vi "Meas_global.vi"() -> ()   [LabVIEW 2022 SP3]
uses:
  Controls/Graph_Type.ctl
  Controls/Post_Process.ctl
  Controls/Trigger_Mode.ctl
  Controls/PWA_Data.ctl
  Controls/Correlation_cluster1.ctl
  Controls/XY_Plot_Cluster.ctl
  Controls/Time_Trace_Cluster.ctl
  Controls/Analysis_info_cluster.ctl
  Controls/Inst_type.ctl
  Controls/Instrument_Array.ctl
  Controls/channelState.ctl
  Controls/Setup.ctl
  Camera Server/Camera enum/Camera resolution.ctl
  File/File Update Cluster.ctl
  Controls/Initial Positions.ctl
  Controls/Initial Info Cluster.ctl
  Gen Trav/Multi_Run_Status.ctl
  Controls/Meas input Cluster.ctl
  Controls/portOrDev.ctl
  Controls/calType.ctl
  Controls/DAQinputType.ctl
panel:
  in  "Tab Control":T1(tab)
  in  "Delay before taking data (ms)":u32
  out "Setup complete?":bool
  in  "Status":T2
  in  "Extra Setup Ch Values":string[](array[string])
  in  "Extra Setup Ch Names":string[](array[string])
  out "Initial Info Cluster":T3[](array[typedef])
  in  "Aborted Setup":bool
  in  "Acquisition Rendezvous":T4
  in  "Time per Block (s)":dbl=100.0 format="%_4f"
  out "MeasurementEndTime":dbl format="%#.2f"
  out "MeasurementStartTime":dbl format="%#.2f"
  out "Nblocks Index":i32
  in  "Current Row Comments":string
  in  "Extra command String":string
  in  "Acquisition Ready":refnum<k4>
  out "Acq ready":bool
  out "Abs Press (mbar)":dbl=1005.0 format="%.2f"
  in  "Start Time of experiment":dbl format="%.2f"
  out "Temp":dbl=20.0 format="%.1f"
  in  "Requested No of blocks":i32
  in  "Post Process":T5
  out "Current Block No":i32
  in  "Remote control":bool
  in  "ADAM Ch Names":string[](array[string])
  in  "Processing last block?":bool
  in  "Averaging time (min)":dbl=6.0 format="%.2f"
  out "Actual Measurement time (min)":dbl=6.0 format="%.2f"
  in  "People to Email":string[](array[string])
  in  "Repeat Measurement?":bool
  in  "Blocks to Skip":i32[](array[numeric])
  in  "Iteration Number":i32
  out "OverrideWait":bool
  in  "setup":T6=enum."Show Setup"
  in  "Zero Offsetting filename":string
  out "svnRevisionOfBinaryData":u32
  out "Flattened data type":enum16{"4.x", "Standard"}(ring)
  out "Time Data was Aquired":dbl format="%.2f"
  in  "Meas Setup filename":string
  in  "Extra Comments":string
  out "ProgRevisionInfo":string
  in  "New Setup String":string
  in  "Pre Setup String":string
  in  "Comments":string
  in  "Raw data file":path
  in  "File":T7(ring)
  in  "Results file":path
  out "Raw data option":enum16{"Save raw data", "Raw data not saved"}(ring)
  out "Start of I16 data (bytes)":i64
  out "Calib file strings":string[](array[string])
  out "Calib type name":string[](array[string])
  out "DAQmx Task Name":refnum<k21>
  in  "TriggerEdge":i32(ring)=10171 items=["Rising"=10280, "Falling"=10171]
  in  "TriggerTTLsource":tag
  in  "Don't Process":bool
  in  "Acquisition Complete?":bool=TRUE
  in  "Measurement.vi Top level?":bool
  in  "Serial Port Aliases":string[][](array[string])
  in  "Called by Zero Instruments.vi":bool
  in  "DAQ Trigger Port":refnum<visa-resource-name>="COM100"
  in  "DAQ Tigger Control?":bool
  in  "Extra ADAM Channel Values":string[](array[string])
  in  "Extra ADAM Channel Names":string[](array[string])
  in  "input terminal configuration":i32(ring)=10106 items=["default"=-1, "RSE"=10083, "NRSE"=10078, "Differential"=10106, "Pseudodifferential"=12529]
  in  "Trigger mode":T8
  in  "Analogue data":enum16{"No Analogue data", "Take Analogue data"}(ring)
  in  "Time Continuous Across Blocks":bool
  in  "output polarity":u16(ring)=1 items=["do not change", "positive", "negative"]
  in  "Over/Under string":string
  in  "Acquisition_Plug_Ins to Run":string[](array[string])
  in  "PWA Data":T9
  in  "stop":bool
  in  "BSA data rate string":string
  in  "LDA data":enum16{"No LDA data", "Take LDA data"}(ring)
  in  "Use  Analogue channel to software sync with LDA":bool
  in  "Blank Output Stats for Chs":i32[](array[numeric])
  out "Initial Probe Positions":T10[](array[typedef])
  out "XYZ Positions From File":dbl[][](array[numeric])
  in  "Template File":path
  in  "Files to Update":T11[](array[typedef])
  in  "Duplicate Chs to correlate":i32[][](array[numeric]) min=0 max=8
  in  "Duplicate_Channels_by_Arithmetic":i32[][](array[numeric]) min=0 max=8
  in  "Create_Derived_Channels_by_Arithmetic":i32[][](array[numeric]) min=0 max=8
  in  "Sub Block Time (s) for Spectra and Auto Corr":dbl=1.0 min=1.0 step=1.0
  in  "Duplicate channels":i32[](array[numeric])
  in  "Smoothing setups":T12(array[cluster]) {"Y axis"."Format" items=["Decimal", "Scientific", "Engineering"]; "Y axis"."Mapping" items=["Linear", "Logarithmic"]; "X axis"."Format" items=["Decimal", "Scientific", "Engineering"]; "X axis"."Mapping" items=["Linear", "Logarithmic"]}
  in  "Cross wire + or -ve":T13(ring)
  in  "Second Graph":T15={"Plot 1"=1, "Plot 2"=3, "Save graph"=0, "Plot Type"=enum."Voltage trace"} {"Save graph" items=["Do not save plot", "Save plot"]; "Plot 2" items=["Nothing", "Velocity1", "Arr time1", "Velocity2", "Arr time2"]; "Plot 1" items=["Nothing", "Velocity1", "Arr time1", "Velocity2", "Arr time2"]}
  in  "First Graph":T15={"Plot 1"=1, "Plot 2"=3, "Save graph"=0, "Plot Type"=enum."Voltage trace"} {"Save graph" items=["Do not save plot", "Save plot"]; "Plot 2" items=["Nothing", "Velocity1", "Arr time1", "Velocity2", "Arr time2"]; "Plot 1" items=["Nothing", "Velocity1", "Arr time1", "Velocity2", "Arr time2"]}
  in  "No of bins in histogram":i32=300
  in  "correlate":i32[][](array[numeric]) min=0 max=8
  in  "Insts for plotting":u16[][](array[ring]) items=["Nothing", "Ref Prop 1", "XW1 1", "XW2 1"]
  out "Unique Times":cluster{"Time (s)":dbl[]}[](array[cluster])
  in  "Time Array Index":i32[](array[numeric])
  out "Fs Used":dbl
  in  "Analysis Info cluster":T16[](array[typedef]) {"Kurt_u" format="%_3g"; "u^4" format="%_3g"; "u^3" format="%_3g"; "Sd Error in Variance" format="%_3g"; "u^2" format="%_3g"; "Sd Error in Mean" format="%_3g"; "U" format="%_3g"; "Sync Delay Time (s)" format="%.4f"; "Total Meas Time (s)" format="%_5g"; "Skew_u" format="%_3g"; "% u'/U" format="%_3g"}
  in  "Time Trace":T20[](array[typedef])
  in  "Autocorrelation":T21[](array[typedef]) {"X array" format="%^_5g"; "Y array" format="%^_5g"}
  in  "Histogram":T21[](array[typedef]) {"X array" format="%^_5g"; "Y array" format="%^_5g"}
  in  "Spectra":T21[](array[typedef]) {"X array" format="%^_5g"; "Y array" format="%^_5g"}
  in  "Confidence Interval (%)":dbl=68.0
  in  "Timescale multiplier for independent samples":dbl=2.0
  in  "Integration threshold (0...1)":dbl=0.25
  in  "Correlation Results":T22[](array[typedef]) {"Time Window (ms)" format="%.2f"; "w^2 Paired" format="%.2f"; "u^2 Paired" format="%.2f"; "u^2w^2" format="%.2f"; "u^3w" format="%.2f"; "uw^3" format="%.2f"; "uw/u'w'" format="%.2f"; "uw^2" format="%.2f"; "u^2w" format="%.2f"; "uw" format="%.2f"}
  in  "Error Messages":string
  out "Diagnostic info":string[][](table)
  out "Vel stat display":string[][](table)
  in  "Error handler Log":string
  in  "Acquiring Pictures":bool
  in  "Webcam Overlay Text":string
  in  "Camera Resolution":T23=1 items=["Low", "Med.", "High", "Max."]
  out "Dynamically Added":T24[](array[typedef]) {"Fs" format="%#_pHz"; "syncDelay" format="%#_gms"; "Ch" min=0 step=1}
  # "The factor to multiply the integral time scale by to correct for a non-zero integration cut-off is now automatically computed using numerical function"
  # "This is the fraction of the correlation peak value at which to cut-off the integration of the correlation function"
  # "(Springer Handbook of Experimental Fluid Mechanics, eqn 23.46)"
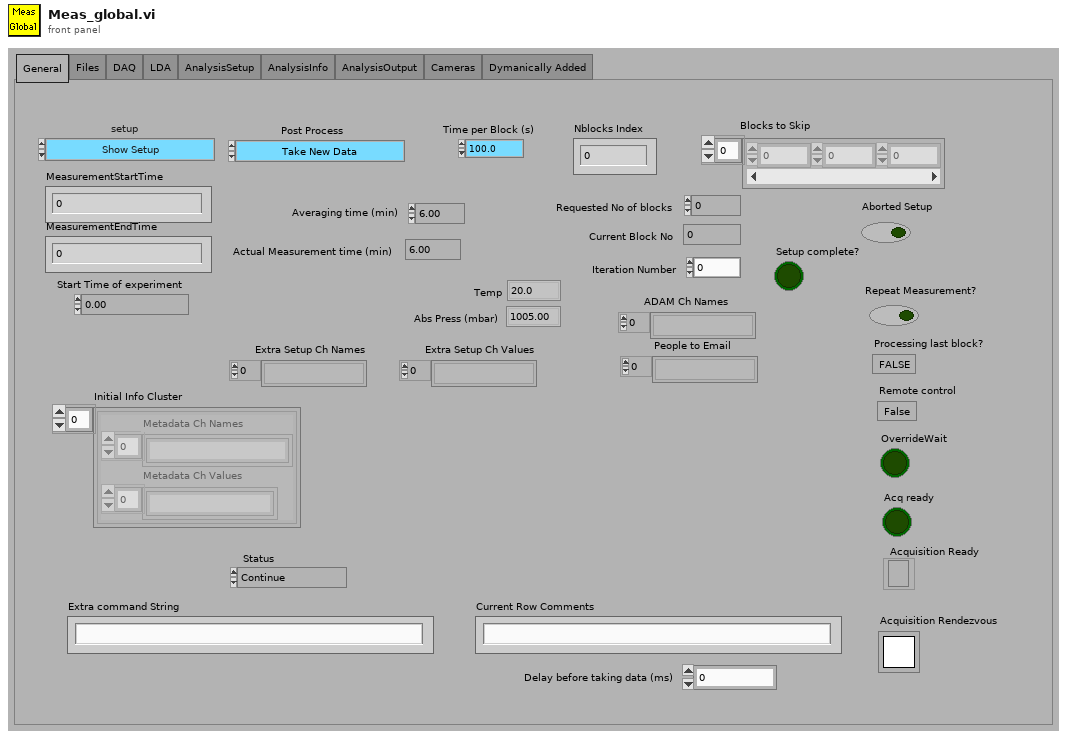
[diagram p1: front panel]
types:
  T1 = enum32{"General", "Files", "DAQ", "LDA", "AnalysisSetup", "AnalysisInfo", "AnalysisOutput", "Cameras", "Dymanically Added"}
  T2 = typedef "Multi_Run_Status.ctl" = enum16{"Continue", "Continue with Error", "Jump to Next Point", "Jump to Next Row", "Jump To Fall Back", "Terminate Run"}
  T3 = typedef "Initial Info Cluster.ctl" = cluster{"Metadata Ch Names":string[], "Metadata Ch Values":string[]}
  T4 = typedef "Rendezvous RefNum" = refnum<k1>
  T5 = typedef "Post_Process.ctl" = enum16{"Take New Data", "Post Process Raw Data File"}
  T6 = typedef "Setup.ctl" = enum16{"Run Program", "Show Setup", "Save Current Setup", "Setup Front Panel"}
  T7 = enum16{"Save no data", "Save data in new files", "Save data in existing files"}
  T8 = typedef "Trigger_Mode.ctl" = enum16{"Free Running", "Start on Trigger", "Trigger Every Block", "Trigger Every Sample"}
  T9 = typedef "PWA_Data.ctl" = enum16{"No PWA Data", "One Ch PWA"}
  T10 = typedef "Initial Positions.ctl" = cluster{"Initial XYZ":sgl[], "Traverse Setup":string, "On Axes":string, "Identity String":string}
  T11 = typedef "File Update Cluster.ctl" = cluster{"File Path":path, "Rows to Add":i32[], "Extra Ch Names":string[], "Extra Ch Values":string[], "Initial Header String":string, "Separation Character":enum16{"Tab", "Comma"}}
  T12 = cluster{"Start Index":i32, "End Index":i32, "Smoothing":enum16{"Linear", "Logarithmic"}, "Number of smoothed estimates":i32, "X axis":cluster{"Mapping":u16, "Format":u16}, "Y axis":cluster{"Mapping":u16, "Format":u16}, "Use Whole Input Array?":bool}[]
  T13 = enum16{"2nd component as calculated", "2nd component multipled by -1"}
  T14 = typedef "Graph_Type.ctl" = enum16{"Show no graph", "Voltage trace", "Velocity trace", "Vel histogram", "Spectrum", "f.E(f) v Log f", "Auto-Corr"}
  T15 = cluster{"Plot 1":u16, "Plot 2":u16, "Save graph":u16, "Plot Type":T14}
  T16 = typedef "Analysis_info_cluster.ctl" = cluster{"Colour":u32, "Inst type":T17, "Inst name":string, "Symbol":string, "Code name":string, "Extra Info":string, "Inst Array":T18, "U":dbl, "u^2":dbl, "u^3":dbl, "u^4":dbl, "Skew_u":dbl, "Kurt_u":dbl, "Sd Error in Mean":dbl, "% u'/U":dbl, "X":dbl, "Y":dbl, "Z":dbl, "Timescale integral Estimate":dbl, "Sd Error in Variance":dbl, "Calib File":path, "Calib Constants":dbl[], "Output Position":bool, "Stats":enum16{"None", "Basic", "Full"}, "Av Sampling Rate":dbl, "Av No of Samples":dbl, "Total Meas Time (s)":dbl, "OrigChName":string, "Max value":dbl, "Min value":dbl, "Req Sample Rate Hz":dbl, "Sync Delay Time (s)":dbl, "Ch No":i16, "Device":string, "Use Latest Calib":bool, "Port":string, "Metadata Ch Names":string[], "Metadata Ch Values":string[], "Label":string, "chState":T19, "Point Drift":dbl, "inputConfig":string}
  T17 = typedef "Inst_type.ctl" = enum16{"Raw voltage", "Raw with zero offsetting", "Propeller anemometer", "Pressure Transducer", "Pitot-static tube", "Hot wire", "Cross wire 1", "Cross wire 2", "Generic Linear", "Generic Polynomial", "Generic BackPoly", "Fast FID", "Thermocouple", "Cold wire", "Pulsed Wire", "LDA Vel", "LDA Tran time", "LDA Arr time", "Microphone"}
  T18 = typedef "Instrument_Array.ctl" = enum16{"PWA", "LDA", "Analogue"}
  T19 = typedef "channelState.ctl" = enum32{"No Selection", "Solo", "Mute"}
  T20 = typedef "Time_Trace_Cluster.ctl" = cluster{"Weighting":dbl[], "Voltage":dbl[], "Eng Values":dbl[]}
  T21 = typedef "XY_Plot_Cluster.ctl" = cluster{"First Name":string, "Second Name":string, "X axis name":string, "Y axis name":string, "X array":dbl[], "Y array":dbl[], "Weighting":dbl[]}
  T22 = typedef "Correlation_cluster1.ctl" = cluster{"U inst":string, "uw":dbl, "u^2w":dbl, "uw^2":dbl, "uw/u'w'":dbl, "W inst":string, "uw^3":dbl, "u^3w":dbl, "u^2w^2":dbl, "Index U":i32, "Index W":i32, "Error info":string[], "Paired Sampling Rate (Hz)":dbl, "u^2 Paired":dbl, "w^2 Paired":dbl, "Time Window (ms)":dbl}
  T23 = typedef "Camera resolution.ctl" = u8
  T24 = typedef "Meas input Cluster.ctl" = cluster{"Type":T17, "Label":string, "DAQ":string, "Port":T25, "Ch":i32, "Cal":path, "calType":T26, "Fs":dbl, "syncDelay":dbl, "chState":T19, "inputConfig":T27}
  T25 = typedef "portOrDev.ctl" = string
  T26 = typedef "calType.ctl" = enum32{"Latest", "Fixed"}
  T27 = typedef "DAQinputType.ctl" = string
diagram:
